vi "RunTestsInCurrentProject.vi"() -> ()   [LabVIEW 2019]
uses:
  TestResult/TestResult.lvclass
  TestRunner/TestRunner.lvclass
  <vilib>/picture/picture.llb/imagedata.ctl
  CodeCoverage/CodeCoverage.lvclass/CodeCoverage.ctl
  ba646177-6d55-4025-8623-73119a03778b.vi
  <vilib>/Analysis/baseanly.llb/Mean (DBL).vi
  ResultTreeListener/ResultTreeListener.lvclass
  C:/Users/de200256/Code/LVUnit/TestListener/TestListener.lvclass
  TestSuite/TestSuite.lvclass
  CodeCoverage/CodeCoverage.lvclass
  <vilib>/Analysis/NI_AALBase.lvlib
  ResultTree/ResultTree.lvclass
panel:
  out "Not Fully Covered VIs":path[](array[path])
  in  "Result Tree":string(tree)
  out "Time for tests [s]":dbl
  out "Total Coverage [%]":dbl format="%0.2f"
  out "Total time [s]":dbl
  out "Count":i32
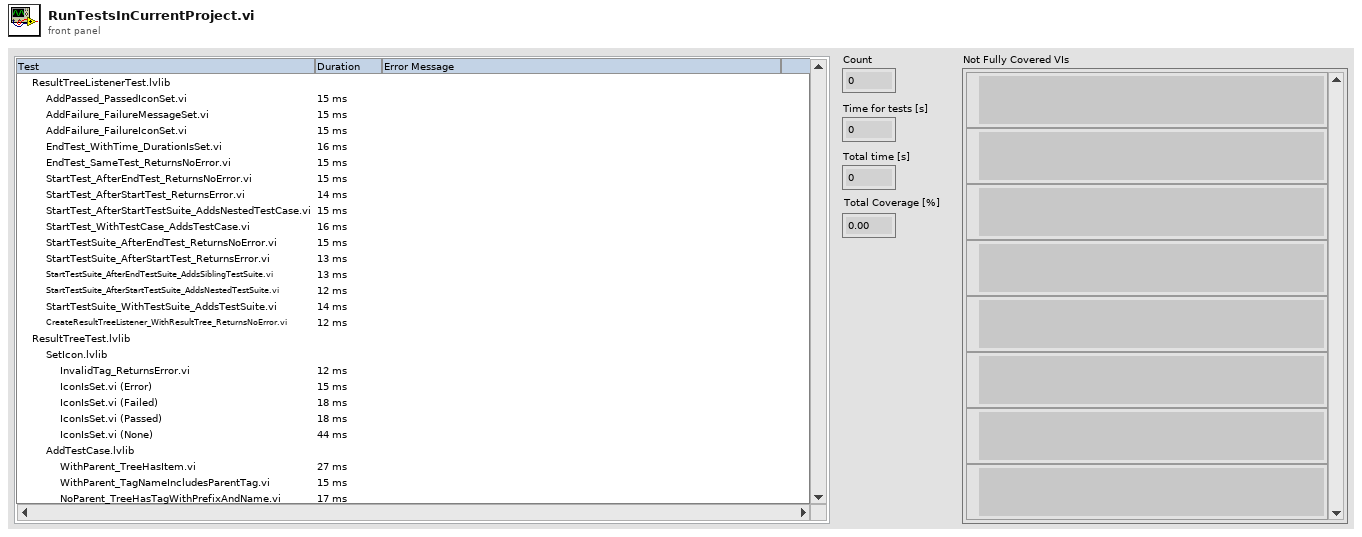
[diagram p1: front panel]
types:
  T1 = typedef "imagedata.ctl" = cluster{"image type":i32, "image depth":i32, "image":u8[], "mask":u8[], "colors":u32[], "Rectangle":cluster{"left":i16, "top":i16, "right":i16, "bottom":i16}}
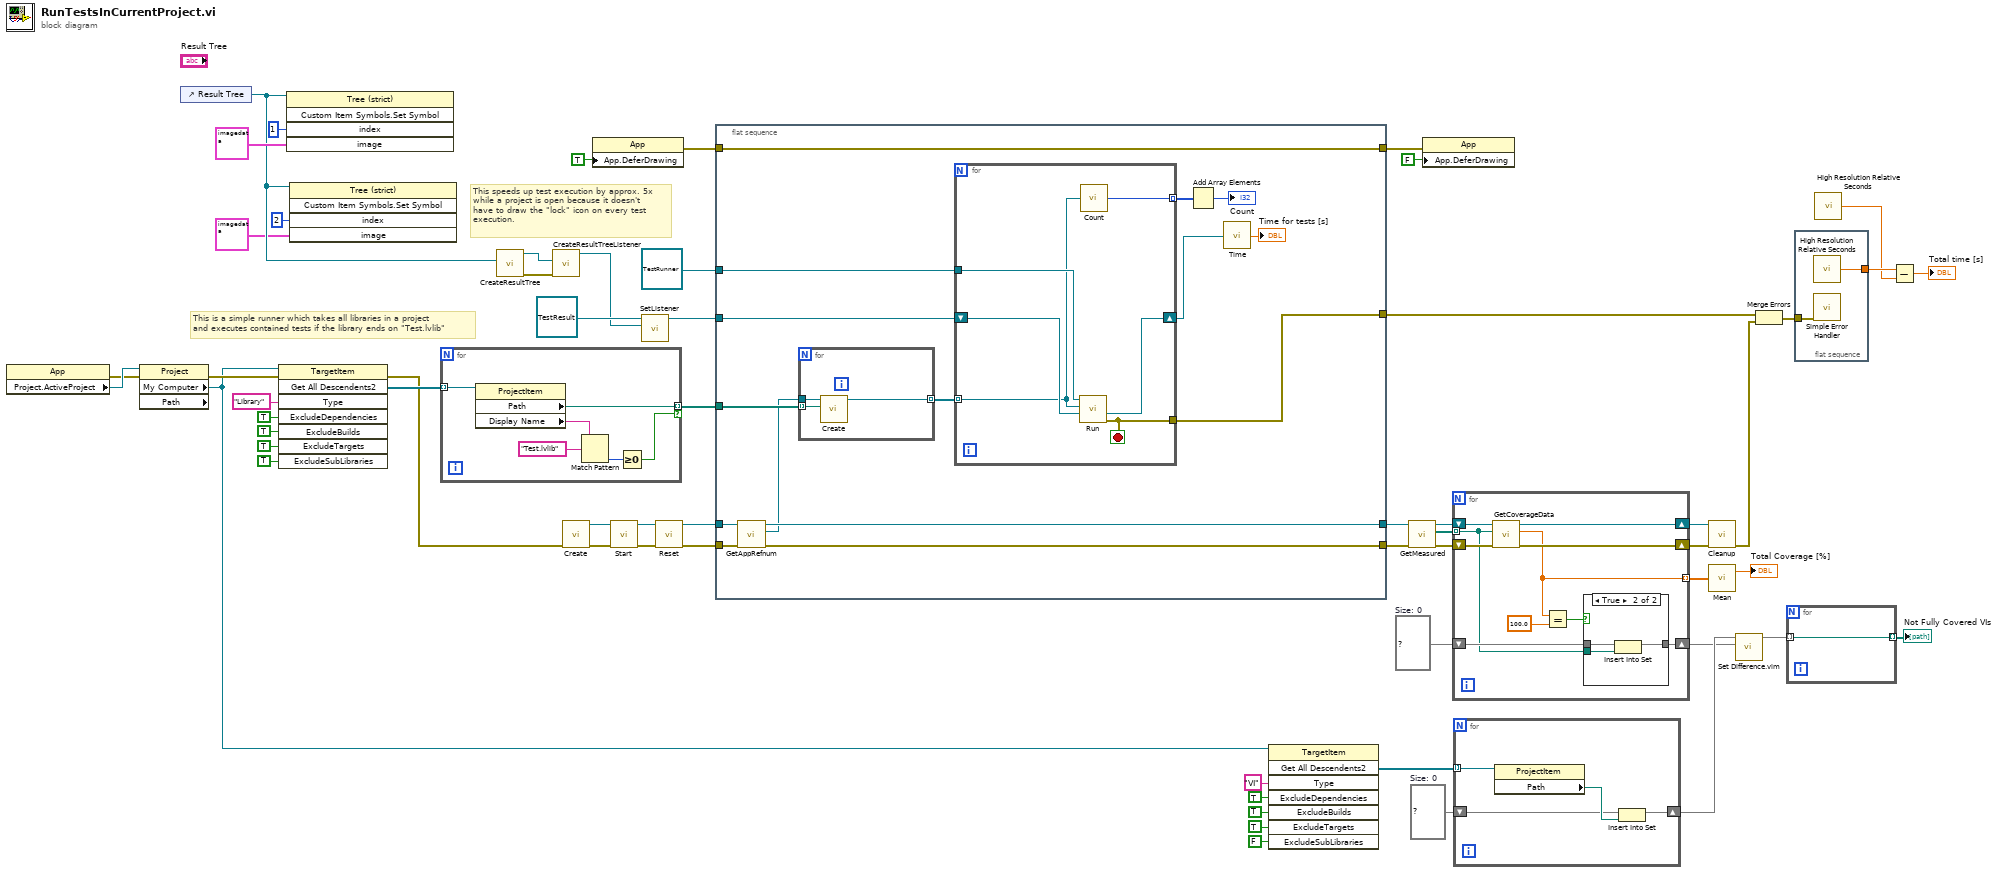
[diagram p0: block diagram]
diagram:
  w5 = set{path} {}  # Size: 0
  w6 = set{path} {}  # Size: 0
  # "This speeds up test execution by approx. 5x\nwhile a project is open because it doesn't\nhave to draw the \"lock\" icon on every test\nexecution."
  # "This is a simple runner which takes all libraries in a project\nand executes contained tests if the library ends on \"Test.lvlib\""
  n1 = property class="App"() -> (error out=w59:errorcluster, "Project.ActiveProject"=w60:refnum<vi>)  [unwired: 2 in, 1 out]
  n2 = property class="Project" props=["My Computer", "Path"](reference=w60, error in=w59) -> (error out=w58:errorcluster, "My Computer"=w13:refnum<vi>)  [unwired: 2 out]
  n3 = control-ref of="Result Tree"() -> (w19:refnum<vi>)
  n4 = invoke class="TargetItem" method="Get All Descendents2"(reference=w13, error in=w58, "Type"="Library", "ExcludeDependencies"=TRUE, "ExcludeBuilds"=TRUE, "ExcludeTargets"=TRUE, "ExcludeSubLibraries"=TRUE) -> (error out=w29:errorcluster, "Get All Descendents2"=w35:refnum<vi>[])  [unwired: 1 in, 6 out]
  n5 = invoke class="Tree (strict)" method="Custom Item Symbols.Set Symbol"(reference=w19, "index"=1 ("Index"), "image"=T1 {"image type"=0, "image depth"=32, "image"=array[1296 elements], "mask"=[0, 0, 0, 0, 0, 0, 0, 0, 63, 255, 0, 0, 63, 255, 0, 0, 63, 255, 0, 0, 63, 255, 0, 0, 63, 255, 0, 0, 63, 255, 0, 0, 63, 255, 0, 0, 63, 255, 0, 0, 63, 255, 0, 0, 63, 255, 0, 0, 63, 255, 0, 0, 63, 255, 0, 0, 63, 255, 0, 0, 63, 255, 0, 0, 0, 0, 0, 0, 0, 0, 0, 0], "colors"=[], "Rectangle"={"left"=0, "top"=0, "right"=18, "bottom"=18}} ("image data")) -> ()  [unwired: 2 in, 5 out]
  n6 = invoke class="Tree (strict)" method="Custom Item Symbols.Set Symbol"(reference=w19, "index"=2 ("Index"), "image"=T1 {"image type"=0, "image depth"=32, "image"=[255, 255, 255, 255, 255, 255, 255, 255, 255, 255, 255, 255, 255, 255, 255, 255, 255, 255, 255, 255, 255, 25, 25, 25, 255, 25, 25, 25, 255, 25, 25, 25, 255, 25, 25, 25, 255, 25, 25, 25, 255, 255, 255, 255, 255, 255, 255, 255, 255, 255, 255, 255, 255, 255, 255, 255, 255, 255, 255, 255, 255, 255, 255, 255, 255, 255, 255, 255, 255, 255, 255, 255, 255, 25, 25, 25, 255, 25, 25, 25, 255, 254, 148, 148, 255, 254, 148, 148, 255, 254, 148, 148, 255, 254, 148, 148, 255, 254, 148, 148, 255, 25, 25, 25, 255, 25, 25, 25, 255, 255, 255, 255, 255, 255, 255, 255, 255, 255, 255, 255, 255, 255, 255, 255, 255, 255, 255, 255, 255, 25, 25, 25, 255, 254, 148, 148, 255, 254, 148, 148, 255, 255, 0, 0, 255, 255, 0, 0, 255, 255, 0, 0, 255, 255, 0, 0, 255, 255, 0, 0, 255, 255, 0, 0, 255, 255, 0, 0, 255, 25, 25, 25, 255, 255, 255, 255, 255, 255, 255, 255, 255, 255, 255, 255, 255, 25, 25, 25, 255, 254, 148, 148, 255, 255, 0, 0, 255, 255, 0, 0, 255, 255, 0, 0, 255, 255, 0, 0, 255, 255, 0, 0, 255, 255, 0, 0, 255, 255, 0, 0, 255, 255, 0, 0, 255, 255, 0, 0, 255, 255, 0, 0, 255, 25, 25, 25, 255, 255, 255, 255, 255, 255, 255, 255, 255, 25, 25, 25, 255, 254, 148, 148, 255, 255, 255, 253, 255, 255, 255, 253, 255, 255, 255, 253, 255, 255, 0, 0, 255, 255, 0, 0, 255, 255, 0, 0, 255, 255, 255, 253, 255, 255, 255, 253, 255, 255, 255, 253, 255, 255, 0, 0, 255, 25, 25, 25, 255, 255, 255, 255, 255, 25, 25, 25, 255, 254, 148, 148, 255, 255, 0, 0, 255, 255, 0, 0, 255, 255, 255, 253, 255, 255, 255, 253, 255, 255, 255, 253, 255, 255, 0, 0, 255, 255, 255, 253, 255, 255, 255, 253, 255, 255, 255, 253, 255, 255, 0, 0, 255, 255, 0, 0, 255, 255, 0, 0, 255, 25, 25, 25, 255, 25, 25, 25, 255, 254, 148, 148, 255, 255, 0, 0, 255, 255, 0, 0, 255, 255, 0, 0, 255, 255, 255, 253, 255, 255, 255, 253, 255, 255, 255, 253, 255, 255, 255, 253, 255, 255, 255, 253, 255, 255, 0, 0, 255, 255, 0, 0, 255, 255, 0, 0, 255, 255, 0, 0, 255, 25, 25, 25, 255, 25, 25, 25, 255, 254, 148, 148, 255, 255, 0, 0, 255, 255, 0, 0, 255, 255, 0, 0, 255, 255, 0, 0, 255, 255, 255, 253, 255, 255, 255, 253, 255, 255, 255, 253, 255, 255, 0, 0, 255, 255, 0, 0, 255, 255, 0, 0, 255, 255, 0, 0, 255, 255, 0, 0, 255, 25, 25, 25, 255, 25, 25, 25, 255, 254, 148, 148, 255, 255, 0, 0, 255, 255, 0, 0, 255, 255, 0, 0, 255, 255, 255, 253, 255, 255, 255, 253, 255, 255, 255, 253, 255, 255, 255, 253, 255, 255, 255, 253, 255, 255, 0, 0, 255, 255, 0, 0, 255, 255, 0, 0, 255, 255, 0, 0, 255, 25, 25, 25, 255, 25, 25, 25, 255, 254, 148, 148, 255, 255, 0, 0, 255, 255, 0, 0, 255, 255, 255, 253, 255, 255, 255, 253, 255, 255, 255, 253, 255, 255, 0, 0, 255, 255, 255, 253, 255, 255, 255, 253, 255, 255, 255, 253, 255, 255, 0, 0, 255, 255, 0, 0, 255, 255, 0, 0, 255, 25, 25, 25, 255, 255, 255, 255, 255, 25, 25, 25, 255, 255, 0, 0, 255, 255, 255, 253, 255, 255, 255, 253, 255, 255, 255, 253, 255, 255, 0, 0, 255, 255, 0, 0, 255, 255, 0, 0, 255, 255, 255, 253, 255, 255, 255, 253, 255, 255, 255, 253, 255, 255, 0, 0, 255, 25, 25, 25, 255, 255, 255, 255, 255, 255, 255, 255, 255, 25, 25, 25, 255, 255, 0, 0, 255, 255, 0, 0, 255, 255, 0, 0, 255, 255, 0, 0, 255, 255, 0, 0, 255, 255, 0, 0, 255, 255, 0, 0, 255, 255, 0, 0, 255, 255, 0, 0, 255, 255, 0, 0, 255, 255, 0, 0, 255, 25, 25, 25, 255, 255, 255, 255, 255, 255, 255, 255, 255, 255, 255, 255, 255, 25, 25, 25, 255, 255, 0, 0, 255, 255, 0, 0, 255, 255, 0, 0, 255, 255, 0, 0, 255, 255, 0, 0, 255, 255, 0, 0, 255, 255, 0, 0, 255, 255, 0, 0, 255, 255, 0, 0, 255, 25, 25, 25, 255, 255, 255, 255, 255, 255, 255, 255, 255, 255, 255, 255, 255, 255, 255, 255, 255, 255, 255, 255, 255, 25, 25, 25, 255, 25, 25, 25, 255, 255, 0, 0, 255, 255, 0, 0, 255, 255, 0, 0, 255, 255, 0, 0, 255, 255, 0, 0, 255, 25, 25, 25, 255, 25, 25, 25, 255, 255, 255, 255, 255, 255, 255, 255, 255, 255, 255, 255, 255, 255, 255, 255, 255, 255, 255, 255, 255, 255, 255, 255, 255, 255, 255, 255, 255, 255, 255, 255, 255, 25, 25, 25, 255, 25, 25, 25, 255, 25, 25, 25, 255, 25, 25, 25, 255, 25, 25, 25, 255, 255, 255, 255, 255, 255, 255, 255, 255, 255, 255, 255, 255, 255, 255, 255, 255, 255, 255, 255], "mask"=[255, 254, 255, 254, 255, 254, 255, 254, 255, 254, 255, 254, 255, 254, 255, 254, 255, 254, 255, 254, 255, 254, 255, 254, 255, 254, 255, 254, 255, 254], "colors"=[], "Rectangle"={"left"=0, "top"=0, "right"=15, "bottom"=15}} ("image data")) -> ()  [unwired: 2 in, 5 out]
  n7 = for {
    tunnel: w35 -> [w66] mode=indexing
    tunnel: [w62] -> w36 mode=indexing if=w61
    n8 = property class="ProjectItem"(reference=w66) -> ("Path"=w62:path, "Display Name"=w63:string)  [unwired: 1 in, 2 out]
    n9 = Match Pattern(string=w63, regular expression="Test.lvlib") -> (offset past match=w64:i32)  [unwired: 1 in, 3 out]
    n10 = Greater Or Equal To 0?(x=w64) -> (x >= 0?=w61:bool)
  }
  n11 = call "CreateResultTree.vi"("Tree Refnum"=w19) -> ("error out"=w14:errorcluster, "ResultTree out"=w16:refnum<class "ResultTree.lvclass">)  [unwired: 9 in]
  n12 = call "CreateResultTreeListener.vi"("error in (no error)"=w14, "ResultTree"=w16) -> ("ResultTreeListener out"=w15:refnum<class "ResultTreeListener.lvclass">)  [unwired: 8 in, 1 out]
  n13 = call "Create.vi"("error in (no error)"=w29) -> ("error out"=w47:errorcluster, "CodeCoverage out"=w32:refnum<class "CodeCoverage.lvclass">)  [unwired: 9 in]
  n14 = property class="App"("App.DeferDrawing"=TRUE ("Application:Defer Drawing")) -> (error out=w26:errorcluster)  [unwired: 2 in, 1 out]
  n15 = call "Start.vi"("error in (no error)"=w47, "CodeCoverage in"=w32) -> ("error out"=w34:errorcluster, "CodeCoverage out"=w31:refnum<class "CodeCoverage.lvclass">)  [unwired: 8 in]
  n16 = call "SetListener.vi"("Listener"=w15, "TestResult in"=refnum<class "TestResult.lvclass"> refnum ("TestResult out")) -> ("TestResult out"=w22:refnum<class "TestResult.lvclass">)  [unwired: 8 in, 1 out]
  n17 = call "Reset.vi"("error in (no error)"=w34, "CodeCoverage in"=w31) -> ("error out"=w33:errorcluster, "CodeCoverage out"=w30:refnum<class "CodeCoverage.lvclass">)  [unwired: 8 in]
  n18 = flat-sequence {
    tunnel: w36 -> [w70]
    tunnel: w22 -> [w81]
    tunnel: [w80] -> w45
    tunnel: refnum<class "TestRunner.lvclass"> refnum ("TestRunner in") -> [w79]
    tunnel: [w73] -> w39
    tunnel: w30 -> [w74]
    tunnel: [w75] -> w48
    tunnel: w33 -> [w76]
    tunnel: [w68] -> w24
    tunnel: w26 -> [w68]
    frame #0 {
      n19 = call "GetAppRefnum.vi"("error in (no error)"=w76, "CodeCoverage in"=w74) -> ("error out"=w75:errorcluster, "App Refnum"=w69:refnum<vi>, "CodeCoverage out"=w73:refnum<class "CodeCoverage.lvclass">)  [unwired: 7 in]
      n20 = for {
        tunnel: w70 -> [w90] mode=indexing
        tunnel: w69 -> [w89]
        tunnel: [w88] -> w67 mode=indexing
        n21 = call "Create.vi"("Path"=w90, "App Refnum (This Application)"=w89) -> ("TestSuite"=w88:refnum<class "TestSuite.lvclass">)  [unwired: 8 in, 1 out]
      }
      n22 = for {
        shift-right: [w86] -> w72
        shift-left: w81 -> [w87]
        tunnel: [w82] -> w80
        tunnel: w79 -> [w85]
        tunnel: [w84] -> w78 mode=indexing
        tunnel: w67 -> [w83] mode=indexing
        stop <- w82 stop-if-true
        n23 = call-dynamic "Run.vi"("TestResult"=w87, "TestSuite"=w83, "TestRunner in"=w85) -> ("error out"=w82:errorcluster, "TestResult out"=w86:refnum<class "TestResult.lvclass">)  [unwired: 6 in, 1 out]
        n24 = call "Count.vi"("TestSuite In"=w83) -> ("Count"=w84:i32)
      }
      n25 = Add Array Elements(numeric array=w78) -> (sum=→"Count":i32)
      n26 = call "Time.vi"("TestResult In"=w72) -> ("Time"=→"Time for tests [s]":dbl)
    }
  }
  n27 = invoke class="TargetItem" method="Get All Descendents2"(reference=w13, "Type"="VI", "ExcludeDependencies"=TRUE, "ExcludeBuilds"=TRUE, "ExcludeTargets"=TRUE, "ExcludeSubLibraries"=FALSE) -> ("Get All Descendents2"=w7:refnum<vi>[])  [unwired: 2 in, 7 out]
  n28 = call "GetMeasured.vi"("error in (no error)"=w48, "CodeCoverage in"=w39) -> ("error out"=w40:errorcluster, "All VIs Measured"=w37:path[], "CodeCoverage out"=w38:refnum<class "CodeCoverage.lvclass">)  [unwired: 7 in]
  n29 = property class="App"(error in=w24, "App.DeferDrawing"=FALSE ("Application:Defer Drawing")) -> ()  [unwired: 1 in, 2 out]
  n30 = for {
    shift-right: [w99] -> w49
    shift-left: w38 -> [w100]
    shift-right: [w97] -> w46
    shift-left: w40 -> [w98]
    tunnel: [w96] -> w42 mode=indexing
    tunnel: w37 -> [w91] mode=indexing
    shift-right: [w93] -> w1
    shift-left: w6 -> [w92]
    n31 = call "GetCoverageData.vi"("error in (no error)"=w98, "VI Path"=w91, "CodeCoverage in"=w100) -> ("error out"=w97:errorcluster, "Coverage Percentage"=w96:dbl, "CodeCoverage out"=w99:refnum<class "CodeCoverage.lvclass">)  [unwired: 6 in]
    n32 = Equal?(x=w96, y=100.0) -> (x = y?=w94:bool)
    n33 = case shown="True" w94 {
      tunnel: [w101 w104] -> w93
      tunnel: w92 -> [w101 w103]
      tunnel: w91 -> [_ w102]
      frame False {
      }
      frame True {
        n34 = Insert Into Set(10:w102, 11:w103) -> (3:w104:set{path})  [unwired: 1 out]
      }
    }
  }
  n35 = for {
    tunnel: w7 -> [w108] mode=indexing
    shift-right: [w106] -> w2
    shift-left: w5 -> [w105]
    n36 = property class="ProjectItem"(reference=w108) -> ("Path"=w107:path)  [unwired: 1 in, 2 out]
    n37 = Insert Into Set(10:w107, 11:w105) -> (3:w106:set{path})  [unwired: 1 out]
  }
  n38 = call "Cleanup.vi"("error in (no error)"=w46, "CodeCoverage in"=w49) -> ("error out"=w43:errorcluster)  [unwired: 9 in]
  n39 = call-poly <vilib>:"Mean.vi"("X"=w42) -> ("mean"=→"Total Coverage [%]":dbl)  [unwired: 1 out]
  n40 = call "Set Difference.vim"("set 2"=w1, "set 1"=w2) -> ("difference"=w4:set{path})  [unwired: 9 in]
  n41 = Merge Errors(w45, w43) -> (w44:errorcluster)
  n42 = for {
    tunnel: w4 -> [w109] mode=indexing
    tunnel: [w109] -> w3 mode=indexing
  }
  "Not Fully Covered VIs" <- w3
  n43 = flat-sequence {
    tunnel: w44 -> [w111]
    tunnel: [w110] -> w52
    frame #0 {
      n44 = call <vilib>:"High Resolution Relative Seconds.vi"() -> ("relative seconds"=w110:dbl)
      n45 = call <vilib>:"Simple Error Handler.vi"("error in (no error)"=w111) -> ()  [unwired: 4 in, 5 out]
    }
  }
  n46 = call <vilib>:"High Resolution Relative Seconds.vi"() -> ("relative seconds"=w51:dbl)
  n47 = Subtract(x=w52, y=w51) -> (x-y=→"Total time [s]":dbl)
